vi "stepper_moveabs_wait.vi"(8 "error in (no error)":errorcluster, 10 "fAbsPos[µm]":sgl min=0 max=4000, 11 "reference":refnum<k7>) -> (0 "error out":errorcluster, 3 "reference out":refnum<k7>)   [LabVIEW 2018]
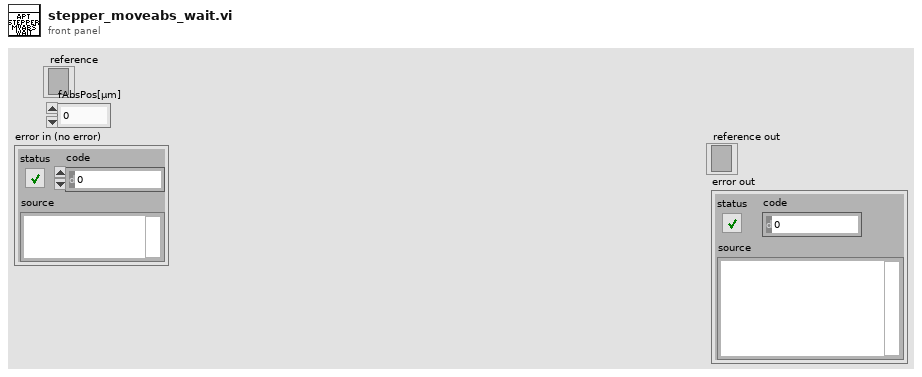
[diagram p1: front panel]
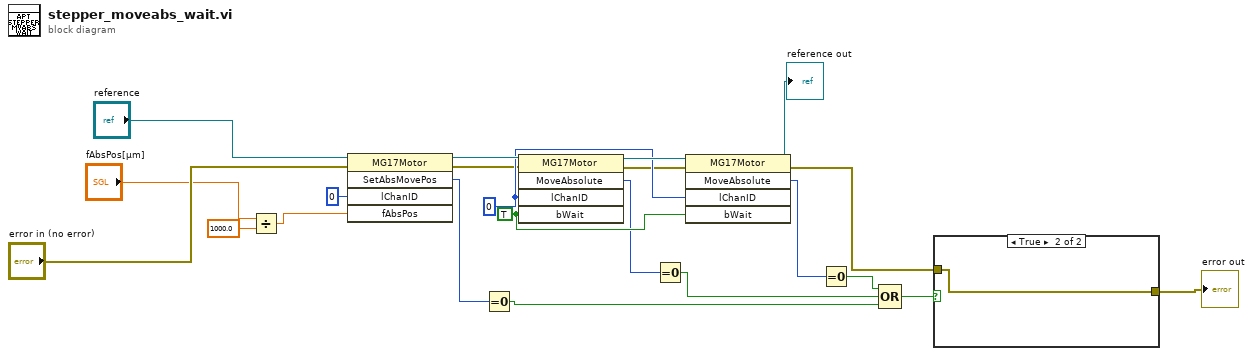
[diagram p0: block diagram]
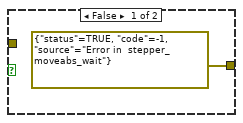
[diagram p2: hidden frame]
diagram:
  w16 = TRUE ("bWait")
  w17 = 0 ("lChanID")
  n1 = Divide(x="fAbsPos[µm]", y=sgl 1000.0) -> (x/y=w13:sgl)
  n2 = invoke class="MG17Motor" method="SetAbsMovePos"(reference="reference", error in="error in (no error)", "lChanID"=0, "fAbsPos"=w13) -> (reference out=w21:refnum<k7>, error out=w3:errorcluster, "SetAbsMovePos"=w11:i32)  [unwired: 1 in, 2 out]
  n3 = Equal To 0?(x=w11) -> (x = 0?=w6:bool)
  n4 = invoke class="MG17Motor" method="MoveAbsolute"(reference=w21, error in=w3, "lChanID"=w17, "bWait"=w16) -> (reference out=w18:refnum<k7>, error out=w2:errorcluster, "MoveAbsolute"=w10:i32)  [unwired: 1 in, 2 out]
  n5 = Equal To 0?(x=w10) -> (x = 0?=w7:bool)
  n6 = invoke class="MG17Motor" method="MoveAbsolute"(reference=w18, error in=w2, "lChanID"=w17, "bWait"=w16) -> (reference out=→"reference out":refnum<k7>, error out=w1:errorcluster, "MoveAbsolute"=w9:i32)  [unwired: 1 in, 2 out]
  n7 = Equal To 0?(x=w9) -> (x = 0?=w8:bool)
  n8 = Compound Arithmetic op=OR(w8, w7, w6) -> (w5:bool)
  n9 = case shown="True" w5 {
    tunnel: [errorcluster {"status"=TRUE, "code"=-1, "source"="Error in  stepper_moveabs_wait"} ("error out") w24] -> w4
    tunnel: w1 -> [_ w24]
    frame False {
    }
    frame True {
    }
  }
  "error out" <- w4
